vi "Search and remove observer.vi"(8 "error in (no error)":errorcluster, 10 "Message in":refnum<class "InformMessage.lvclass">, 11 "Chat in":refnum<class "Chat.lvclass">) -> (0 "error out":errorcluster, 3 "Chat out":refnum<class "Chat.lvclass">)   [LabVIEW 2012, in "Chat.lvclass"]
uses:
  Chat.lvclass
  <vilib>/Distrio/Murmex/InformMessage/InformMessage.lvclass
  Chat.lvclass/Chat.ctl
  <vilib>/Distrio/Murmex/Message/Message.lvclass
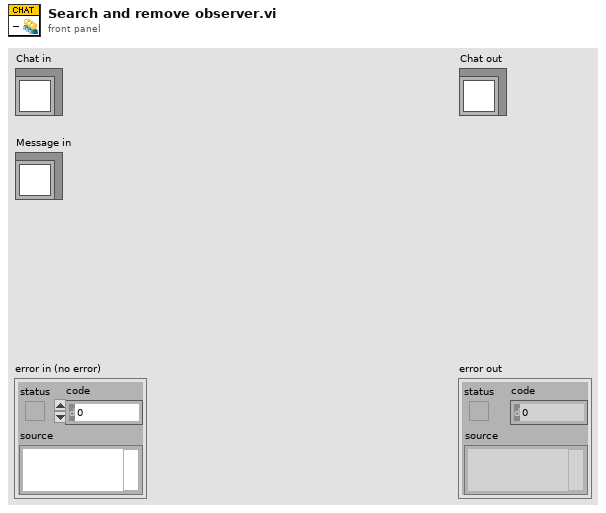
[diagram p1: front panel]
types:
  T1 = typedef "Chat.lvclass/observers_cluster.ctl" = cluster{"id":string, "writing":bool}
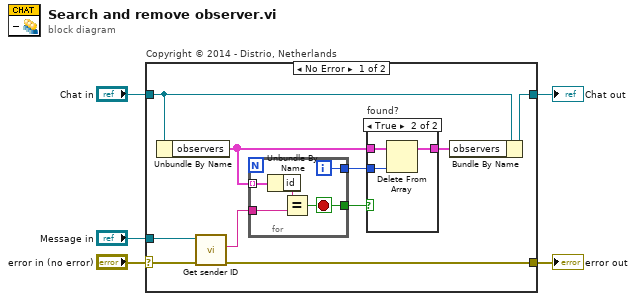
[diagram p0: block diagram]
diagram:
  n1 = case "Copyright © 2014 - Distrio, Netherlands" shown="No Error" "error in (no error)" {
    selector: "error in (no error)" -> [w15 w26]
    tunnel: [w14 w26] -> w2
    tunnel: [w8 w25] -> w1
    tunnel: "Chat in" -> [w9 w25]
    tunnel: "Message in" -> [w7 _]
    frame No Error {
      n2 = Unbundle By Name(w9) -> ("observers"=w12:T1[])
      n3 = call <vilib>:"Get sender ID.vi"("error in (no error)"=w15, "Message in"=w7) -> ("error out"=w14:errorcluster, "sender"=w11:string)  [unwired: 7 in, 1 out]
      n4 = for {
        tunnel: w12 -> [w24] mode=indexing
        tunnel: w11 -> [w22]
        tunnel: [w21] -> w13
        tunnel: [w20] -> w6
        i -> [w20]
        stop <- w21 stop-if-true
        n5 = Unbundle By Name(w24) -> ("id"=w23:string)
        n6 = Equal?(x=w23, y=w22) -> (x = y?=w21:bool)
      }
      n7 = case "found?" shown="True" w13 {
        tunnel: w12 -> [w16 w19]
        tunnel: [w16 w18] -> w10
        tunnel: w6 -> [_ w17]
        frame False {
        }
        frame True {
          n8 = Delete From Array(array=w19, index=w17) -> (array with subset deleted=w18:T1[])  [unwired: 1 in, 1 out]
        }
      }
      n9 = Bundle By Name(cluster=w9, "observers"=w10) -> (w8:refnum<class "Chat.lvclass">)
    }
    frame Error {
    }
  }
  "error out" <- w2
  "Chat out" <- w1
